vi "Update Balance API.vi"(8 "Error In":errorcluster, 11 "Update":cluster{"Account Number":i32, "Udpate":dbl}) -> (0 "error in (no error)":errorcluster)   [LabVIEW 2019, in "Configuration Database.lvlib"]
doc: "This method receives an account number and update balance information and queues a message to database module to update the balance of the desired account."
uses:
  Configuration Database.lvlib
  Architecture/Typedefs/Enum_Module_Name.ctl
  Architecture/Architecture.lvlib
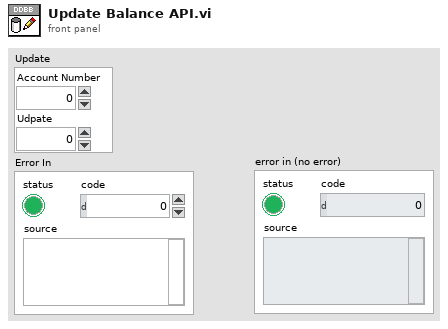
[diagram p1: front panel]
types:
  T1 = typedef "Architecture.lvlib/Enum_Module_Name.ctl" = enum16{"Configuration", "Error_Handler", "Log", "Database", "Controller", "User Console", "Display Console", "Sensor Interface"}
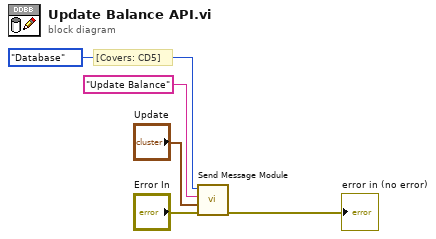
[diagram p0: block diagram]
diagram:
  # "[Covers: CD5]"
  n1 = call "Send Message Module.vi"("Error In"="Error In", "Data"="Update", "Message"="Update Balance", "Target ModuleName In"=Enum_Module_Name."Database") -> ("error in (no error)"=→"error in (no error)":errorcluster)  [unwired: 7 in]
